vi "System Actor Initialize.vi"(5 "Launching":bool=TRUE, 7 "Auto Dispose Ref":bool, 8 "error in (no error)":errorcluster, 10 "Root Actor Address":refnum<class "Mail Strategy.lvclass">, 11 "System Actor in":refnum<class "System Actor.lvclass">) -> (0 "error out":errorcluster, 2 "VI Refnum":refnum<vi>, 3 "System Actor out":refnum<class "System Actor.lvclass">)   [LabVIEW 2024, in "System Actor.lvclass"]
uses:
  System Actor.lvclass
  Messenger/Mail Strategy/Mail Strategy.lvclass
  <vilib>/Utility/config.llb/NI_LVConfig.lvlib
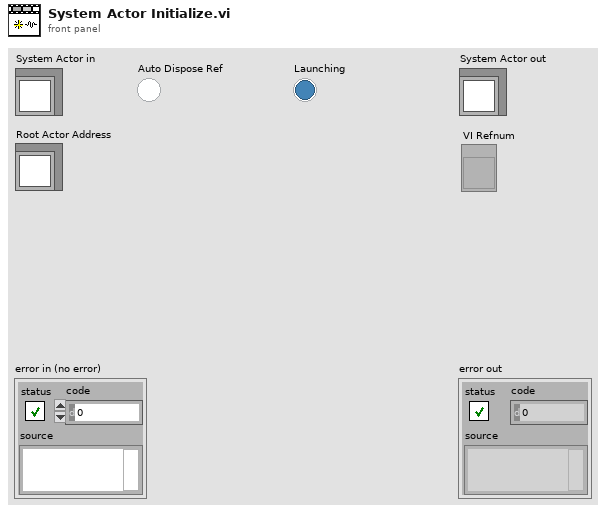
[diagram p1: front panel]
types:
  T1 = typedef "NI_LVConfig.lvlib/Config Data RefNum.ctl" = refnum<k1>
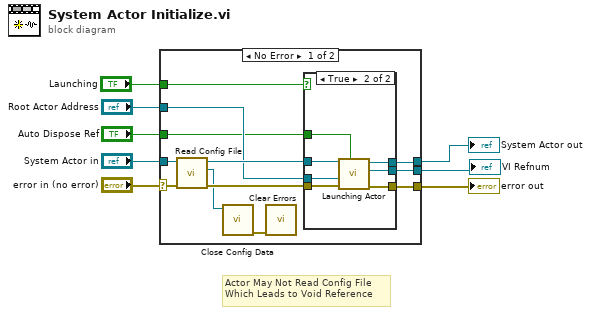
[diagram p0: block diagram]
diagram:
  # "Actor May Not Read Config File\nWhich Leads to Void Reference"
  n1 = case shown="No Error" "error in (no error)" {
    selector: "error in (no error)" -> [w19 w31]
    tunnel: [w15 w31] -> w7
    tunnel: [w16 w30] -> w5
    tunnel: "System Actor in" -> [w20 w30]
    tunnel: [w14 _] -> w4
    tunnel: "Root Actor Address" -> [w13 _]
    tunnel: "Auto Dispose Ref" -> [w11 _]
    tunnel: "Launching" -> [w10 _]
    frame No Error {
      n2 = call-dynamic "Read Config File.vi"("error in (no error)"=w19, "System Actor in"=w20) -> ("error out"=w17:errorcluster, "Ref"=w12:T1, "System Actor out"=w18:refnum<class "System Actor.lvclass">)  [unwired: 7 in]
      n3 = call <vilib>:"Close Config Data.vi"("refnum"=w12) -> ("error out"=w9:errorcluster)  [unwired: 9 in, 1 out]
      n4 = call <vilib>:"Clear Errors.vi"("error in (no error)"=w9) -> ()  [unwired: 5 in, 2 out]
      n5 = case shown="True" w10 {
        tunnel: w18 -> [w22 w29]
        tunnel: w17 -> [w21 w28]
        tunnel: [w22 w27] -> w16
        tunnel: [w21 w26] -> w15
        tunnel: [_ w25] -> w14
        tunnel: w13 -> [_ w24]
        tunnel: w11 -> [_ w23]
        frame False {
        }
        frame True {
          n6 = call-dynamic "Launching Actor.vi"("Auto Dispose Ref"=w23, "error in (no error)"=w28, "Root Actor Address"=w24, "System Actor in"=w29) -> ("error out"=w26:errorcluster, "VI Refnum"=w25:refnum<vi>, "System Actor out"=w27:refnum<class "System Actor.lvclass">)  [unwired: 5 in]
        }
      }
    }
    frame Error {
    }
  }
  "error out" <- w7
  "System Actor out" <- w5
  "VI Refnum" <- w4
